vi "Default Instrument Setup.vi"(8 "error in (no error)":errorcluster, 11 "VISA resource name":refnum<visa-resource-name>) -> (0 "error out":errorcluster, 3 "VISA resource name out":refnum<visa-resource-name>)   [LabVIEW 2024, in "Lake Shore 336.lvlib"]
doc: "This Utility VI sends a default command string to the instrument whenever a new VISA session is opened, or the instrument is reset. Use this VI as a subVI for the <B>Initialize</B> and <B>Reset</B> VIs. Altering this VI could cause these two VIs to operate incorrectly."
uses:
  Lake Shore 336.lvlib
  Instance           1 32Saved   Default Instrument Setup .vi
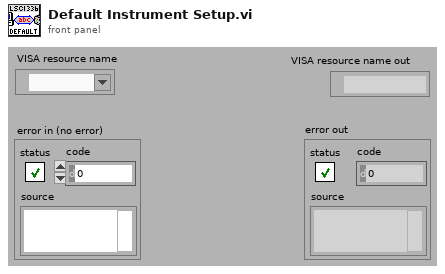
[diagram p1: front panel]
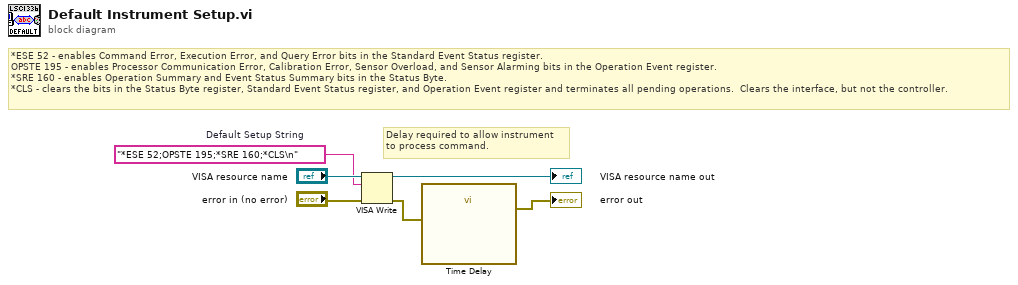
[diagram p0: block diagram]
diagram:
  w4 = "*ESE 52;OPSTE 195;*SRE 160;*CLS\n"  # Default Setup String
  # "*ESE 52 - enables Command Error, Execution Error, and Query Error bits in the Standard Event Status register.\nOPSTE 195 - enables Processor Communication Error, Calibration Error, Sensor Overload, and Sensor Alarming bits in the Operation Event register.\n*SRE 160 - enables Operation Summary and Event Status Summary bits in the Status Byte.\n*CLS - clears the bits in the Status Byte register, Standard Event Status register, and Operation Event register and terminates all pending operations.  Clears the interface, but not the controller."
  # "Delay required to allow instrument\nto process command."
  n1 = VISA Write(VISA resource name="VISA resource name", write buffer=w4, error in (no error)="error in (no error)") -> (VISA resource name out=→"VISA resource name out":refnum<visa-resource-name>, error out=w2:errorcluster)  [unwired: 1 out]
  n2 = call "Time Delay"("error in (no error)"=w2) -> ("error out"=→"error out":errorcluster)  [unwired: 10 in]
